vi "ELVIS III v1.0 AI Continuous Config Bank B.vi"(0 "AI (Continuous) Channels FPGA Reference":T1, 1 "Bank Config":u8[](array[numeric]), 2 "Count (tick/s)":u32, 3 "error in (no error)":errorcluster) -> (10 "error out":errorcluster)   [LabVIEW 2021]
uses:
  <vilib>/myRIO/Common/Instrument Driver Framework/ELVIS III v1.0/AI Block/typedefs/ELVIS III AI Block Channels FPGA Reference.ctl
  <vilib>/rvi/errors/niLvFpgaAdjustHostInterfaceError.vi
  <vilib>/rvi/interface/nirviReadWriteControl/nirviReadWriteControl.xnode
  <vilib>/rvi/interface/Simulation/niFpgaSimulationCallBeginRW.vi
  NiFpgaLv.dll
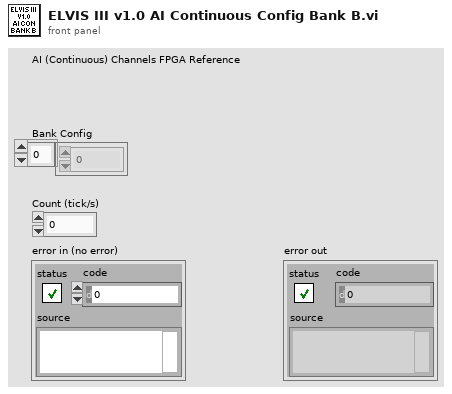
[diagram p1: front panel]
types:
  T1 = typedef "ELVIS III AI Block Channels FPGA Reference.ctl" = refnum<k20>
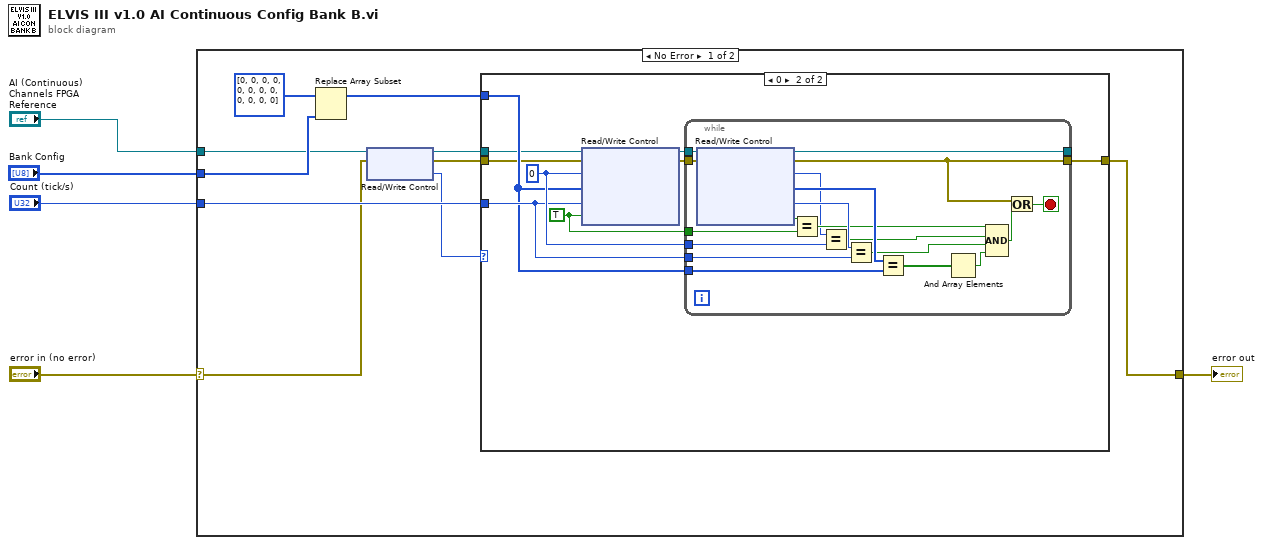
[diagram p0: block diagram]
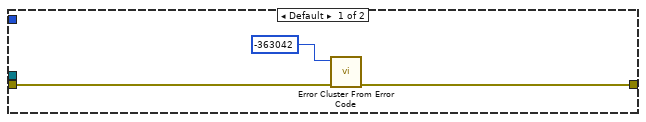
[diagram p2: hidden frame]
diagram:
  n1 = case shown="No Error" "error in (no error)" {
    selector: "error in (no error)" -> [w8 w47]
    tunnel: "AI (Continuous) Channels FPGA Reference" -> [w10 _]
    tunnel: "Count (tick/s)" -> [w13 _]
    tunnel: "Bank Config" -> [w14 _]
    tunnel: [w11 w47] -> w1
    frame No Error {
      n2 = Replace Array Subset(array=u8[] [0, 0, 0, 0, 0, 0, 0, 0, 0, 0, 0, 0] ("AI.A.CNFG"), new element=w14) -> (w12:u8[])  [unwired: 1 in]
      n3 = xnode "Read/Write Control"("FPGA VI Reference In"=w10, "error in"=w8) -> ("FPGA VI Reference Out"=w9:T1, "error out"=w7:errorcluster, "AI.B.CNT"=w6:u8)
      n4 = case shown="0" w6 {
        tunnel: w13 -> [_ w23]
        tunnel: w12 -> [_ w22]
        tunnel: [w16 w21] -> w11
        tunnel: w9 -> [_ w20]
        tunnel: w7 -> [w17 w19]
        frame Default {
          n5 = call <vilib>:"Error Cluster From Error Code.vi"("error in (no error)"=w17, "error code (0)"=-363042) -> ("error out"=w16:errorcluster)  [unwired: 7 in]
        }
        frame 0 {
          w25 = TRUE ("AI.A.DMA_ENA")
          w24 = u8 0 ("AI.A.CNT")
          n6 = xnode "Read/Write Control"("FPGA VI Reference In"=w20, "error in"=w19, "AI.B.CNT"=w24, "AI.B.CNFG"=w22, "AI.B.CNTR"=w23, "AI.B.DMA_ENA"=w25) -> ("FPGA VI Reference Out"=w26:T1, "error out"=w27:errorcluster)
          n7 = while {
            tunnel: w26 -> [w46]
            tunnel: w27 -> [w45]
            tunnel: [w44] -> _
            tunnel: [w36] -> w21
            tunnel: w22 -> [w34]
            tunnel: w23 -> [w42]
            tunnel: w24 -> [w40]
            tunnel: w25 -> [w31]
            stop <- w35 stop-if-true
            n8 = xnode "Read/Write Control"("FPGA VI Reference In"=w46, "error in"=w45) -> ("FPGA VI Reference Out"=w44:T1, "error out"=w36:errorcluster, "AI.B.CNT"=w29:u8, "AI.B.CNFG"=w43:u8[], "AI.B.CNTR"=w41:u32, "AI.B.DMA_ENA"=w32:bool)
            n9 = Equal?(x=w32, y=w31) -> (x = y?=w30:bool)
            n10 = Equal?(x=w29, y=w40) -> (x = y?=w39:bool)
            n11 = Equal?(x=w41, y=w42) -> (x = y?=w38:bool)
            n12 = Equal?(x=w43, y=w34) -> (x = y?=w28:bool[])
            n13 = And Array Elements(Boolean array=w28) -> (logical AND=w33:bool)
            n14 = Compound Arithmetic op=AND(w30, w39, w38, w33) -> (w37:bool)
            n15 = Or(x=w36, y=w37) -> (x .or. y?=w35:bool)
          }
        }
      }
    }
    frame Error {
    }
  }
  "error out" <- w1
